vi "FrequencyMeasurement.vi"(10 "Command Echo":u8[](array[numeric]), 11 "Scalar":dbl) -> (1 "Waveform Graph 2":u16[](graph), 2 "Tuner Recommendation":string, 3 "detected frequency":dbl)   [LabVIEW 2019]
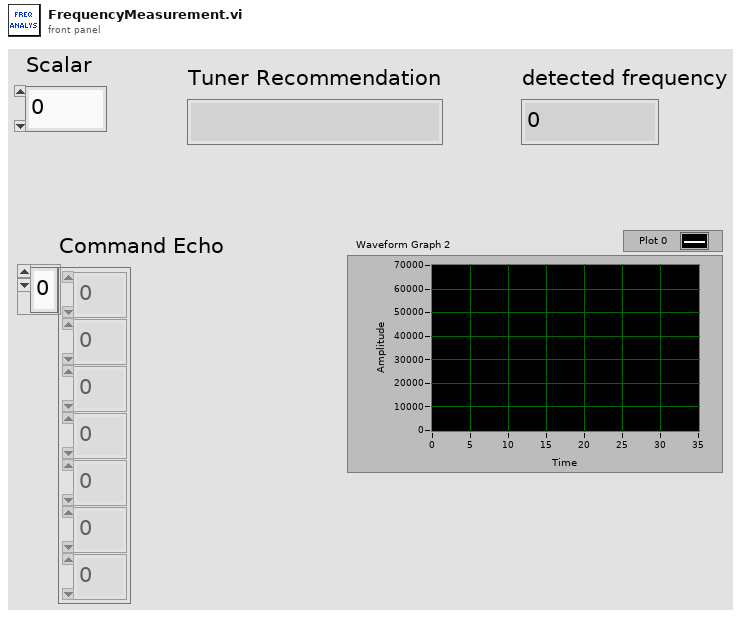
[diagram p1: front panel]
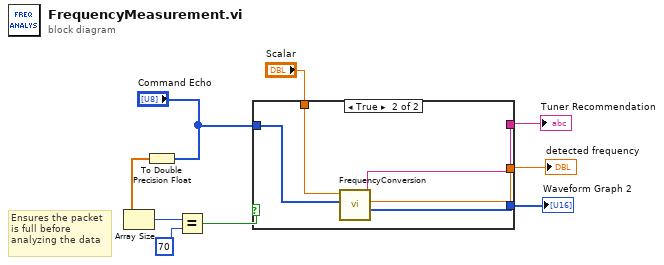
[diagram p0: block diagram]
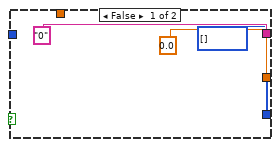
[diagram p2: hidden frame]
diagram:
  # "Ensures the packet\nis full before\nanalyzing the data"
  n1 = To Double Precision Float(number="Command Echo") -> (double precision float=w2:dbl[])
  n2 = Array Size(array=w2) -> (size(s)=w4:i32)
  n3 = Equal?(x=w4, y=70 ("x")) -> (x = y?=w6:bool)
  n4 = case shown="True" w6 {
    tunnel: "Command Echo" -> [_ w17]
    tunnel: "Scalar" -> [_ w16]
    tunnel: ["0" ("Tuner Recommendation") w15] -> w8
    tunnel: [0.0 ("detected frequency") w14] -> w9
    tunnel: [u16[] [] ("Waveform Graph") w13] -> w1
    frame False {
    }
    frame True {
      n5 = call "FrequencyConversion.vi"("Command Echo"=w17, "Scalar"=w16) -> ("Waveform Graph"=w13:u16[], "detected frequency"=w14:dbl, "Tuner Recommendation"=w15:string)  [unwired: 7 in]
    }
  }
  "detected frequency" <- w9
  "Tuner Recommendation" <- w8
  "Waveform Graph 2" <- w1
